vi "sendBLMessage.vi"(5 "blMessageData":u8[](array[numeric]), 7 "blMessage":T2=520224768 items=["LM_API_UPD_PING"=520224768, "LM_API_UPD_DOWNLOAD"=520224832, "LM_API_UPD_SEND_DATA"=520224896, "LM_API_UPD_RESET"=520224960, "LM_API_UPD_ACK"=520225024, "LM_API_UPD_REQUEST"=520225152], 8 "Error in":errorcluster {"code" format="%.0x"}, 11 "ObjHandle in":T1) -> (0 "Error out":errorcluster {"code" format="%.0x"}, 3 "ObjHandle out":T1)   [LabVIEW 2017]
uses:
  LM_API_UPD.ctl
  <vilib>/nican/nican.llb/xobjhandle.ctl
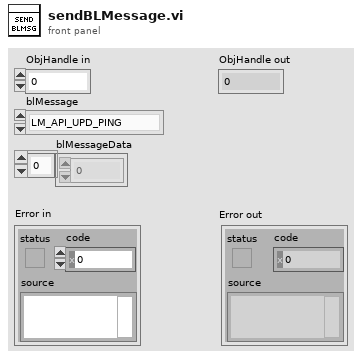
[diagram p1: front panel]
types:
  T1 = typedef "xobjhandle.ctl" = u32
  T2 = typedef "LM_API_UPD.ctl" = u32
  T3 = cluster{dbl, "blMessage":T2, "IsRemote":u8, i32, "blMessageData":u8[]}
  T4 = cluster{dbl, "blMessage":T2, "IsRemote":u8, i32, "blMessageData":u8[]}[]
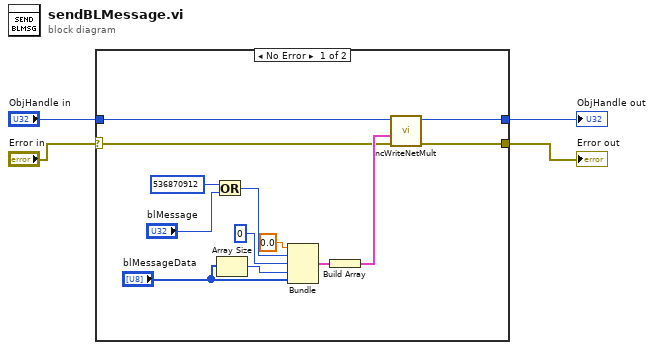
[diagram p0: block diagram]
diagram:
  n1 = case shown="No Error" "Error in" {
    selector: "Error in" -> [w6 w18]
    tunnel: "ObjHandle in" -> [w8 w19]
    tunnel: [w7 w19] -> w3
    tunnel: [w5 w18] -> w1
    frame No Error {
      n2 = Or(x=u32 536870912 ("y"), y="blMessage") -> (x .or. y?=w12:T2)
      n3 = Array Size(array="blMessageData") -> (size(s)=w10:i32)
      n4 = Bundle(0.0, "blMessage"=w12, "IsRemote"=u8 0, w10, "blMessageData"="blMessageData") -> (w15:T3)  [unwired: 1 in]
      n5 = Build Array(w15) -> (w14:T4)
      n6 = call <vilib>:"ncWriteNetMult.vi"("Error in"=w6, "Data"=w14, "ObjHandle in"=w8) -> ("Error out"=w5:errorcluster, "ObjHandle out"=w7:T1)  [unwired: 7 in]
    }
    frame Error {
    }
  }
  "ObjHandle out" <- w3
  "Error out" <- w1
